vi "Conn Modify Reference Count.vi"(6 "error in (no error)":errorcluster, 7 "operation":enum16{"Add", "Subtract"}(ring), 8 "object":enum16{"Recordset", "Command"}(ring), 9 "connection reference":T1) -> (0 "error out":errorcluster, 3 "connection reference out":T1)   [LabVIEW 2013, in "NI_Database_API_64.lvlib"]
doc: "Modifies the contents of a <B>Connection</B> object. The number of objects (recordset or command) is modified according to the operation value (add or subtract)."
uses:
  NI_Database_API_64.lvlib
  Conn ObjectReference.ctl
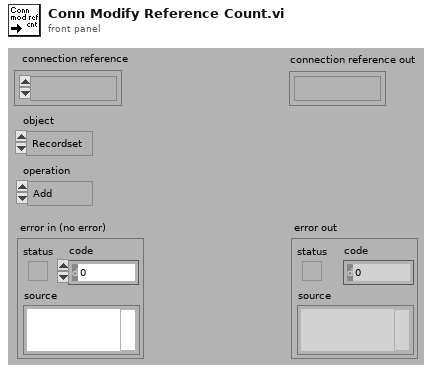
[diagram p1: front panel]
types:
  T1 = typedef "NI_Database_API_64.lvlib/Conn ObjectReference.ctl" = refnum<k1>
  T2 = typedef "NI_Database_API_64.lvlib/Conn DataMembers.ctl" = cluster{"ADODB._Connection":refnum<k7>, "recordset objects":i32, "command objects":i32}
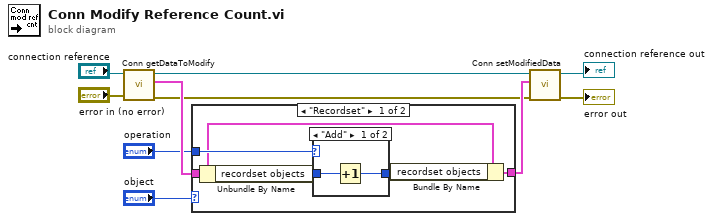
[diagram p0: block diagram]
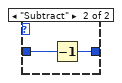
[diagram p2: hidden frame]
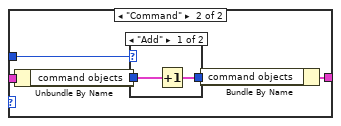
[diagram p3: hidden frame]
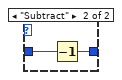
[diagram p4: hidden frame]
diagram:
  n1 = call "Conn getDataToModify.vi"("error in (no error)"="error in (no error)", "connection reference"="connection reference") -> ("error out"=w1:errorcluster, "data"=w4:T2, "connection reference out"=w6:T1)  [unwired: 2 in, 1 out]
  n2 = case shown="\"Recordset\"" "object" {
    tunnel: w4 -> [w12 w21]
    tunnel: "operation" -> [w15 w24]
    tunnel: [w11 w20] -> w2
    frame "Recordset" {
      n3 = Unbundle By Name(w12) -> ("recordset objects"=w14:i32)
      n4 = case shown="\"Add\"" w15 {
        tunnel: w14 -> [w17 w19]
        tunnel: [w16 w18] -> w13
        frame "Add" {
          n5 = Increment(x=w17) -> (x+1=w16:i32)
        }
        frame "Subtract" {
          n6 = Decrement(x=w19) -> (x-1=w18:i32)
        }
      }
      n7 = Bundle By Name(cluster=w12, "recordset objects"=w13) -> (w11:T2)
    }
    frame "Command" {
      n8 = Unbundle By Name(w21) -> ("command objects"=w23:i32)
      n9 = case shown="\"Add\"" w24 {
        tunnel: w23 -> [w26 w28]
        tunnel: [w25 w27] -> w22
        frame "Add" {
          n10 = Increment(x=w26) -> (x+1=w25:i32)
        }
        frame "Subtract" {
          n11 = Decrement(x=w28) -> (x-1=w27:i32)
        }
      }
      n12 = Bundle By Name(cluster=w21, "command objects"=w22) -> (w20:T2)
    }
  }
  n13 = call "Conn setModifiedData.vi"("error in (no error)"=w1, "data"=w2, "connection reference"=w6) -> ("error out"=→"error out":errorcluster, "connection reference out"=→"connection reference out":T1)  [unwired: 3 in]
